vi "Agilent 3446X Series Acquire Single.vi"(2 "error in (no error)":errorcluster, 3 "Measurement Function (10: Voltage DC)":i32(ring)=2 items=["Continuity", "Current AC", "Current DC", "Diode", "Frequency", "Resistance 4-wire", "Period", "Resistance 2-wire", "Temperature", "Voltage AC", "Voltage DC", "Voltage DC Ratio"], 4 "VISA resource name":refnum<visa-resource-name>="USB0::0x0957::0x1A07::MY53207731::INSTR") -> (0 "error out":errorcluster caption="错误输出", 1 "Measurement":dbl)   [LabVIEW 2015]
doc: "This example shows how to configure a measurement and take a reading."
uses:
  Agilent 3446X Series1.lvlib
  Public/Data/Read (Single Point)1.vi
panel:
  in  "Manual Range (1)":dbl=1.0
  in  "Auto Range (T: Enable)":bool=TRUE
  in  "Absolute Resolution (1E-6)":dbl=1e-06
  # "(c) 2013 National Instruments.  ALL RIGHTS RESERVED."
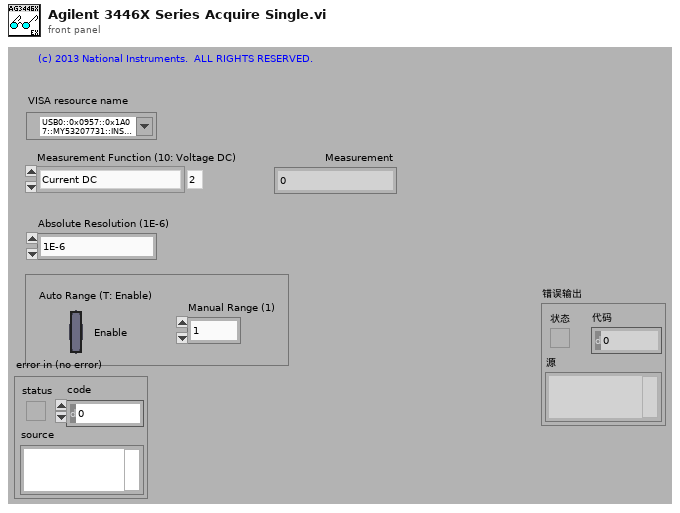
[diagram p1: front panel]
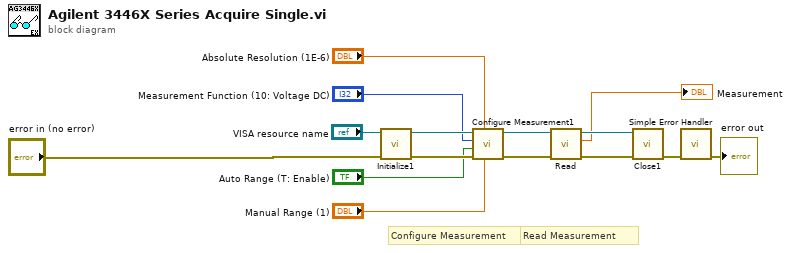
[diagram p0: block diagram]
diagram:
  # "Read Measurement"
  # "Configure Measurement"
  n1 = call "Initialize1.vi"("error in (no error)"="error in (no error)", "VISA resource name"="VISA resource name") -> ("error out"=w13:errorcluster, "VISA resource name out"=w14:refnum<visa-resource-name>)  [unwired: 3 in, 5 out]
  n2 = call "Configure Measurement1.vi"("Manual Range (1)"="Manual Range (1)", "Absolute Resolution (1E-6)"="Absolute Resolution (1E-6)", "error in (no error)"=w13, "Auto Range (T: Enable)"="Auto Range (T: Enable)", "Measurement Function (10: Voltage DC)"="Measurement Function (10: Voltage DC)", "VISA resource name"=w14) -> ("error out"=w9:errorcluster, "VISA resource name out"=w10:refnum<visa-resource-name>)  [unwired: 4 out]
  n3 = call-poly "Read.vi"("error in (no error)"=w9, "VISA resource name"=w10) -> ("error out"=w12:errorcluster, "Measurement"=→"Measurement":dbl, "VISA resource name out"=w11:refnum<visa-resource-name>)  [unwired: 7 out]
  n4 = call "Close1.vi"("error in (no error)"=w12, "VISA resource name"=w11) -> ("error out"=w15:errorcluster)  [unwired: 9 out]
  n5 = call <vilib>:"Simple Error Handler.vi"("error in (no error)"=w15) -> ("error out"=→"error out":errorcluster)  [unwired: 1 in, 7 out]
